vi "Speed Benchmark.vi"() -> ()   [LabVIEW 2015]
uses:
  <vilib>/Platform/TimedLoop/XDataNode/timing_clust.ctl
  <vilib>/Platform/TimedLoop/XDataNode/nitl_modes.ctl
  <vilib>/Platform/TimedLoop/XDataNode/wakeup.ctl
  <vilib>/rvi/Emulation/niFpgaSctlEmulationGetInTimedLoop.vi
  <vilib>/rvi/Emulation/niFpgaEmulationReportErrorSimple.vi
  <vilib>/rvi/Emulation/niFpgaGetClockAttributes.vi
  <vilib>/rvi/Emulation/niFpgaCriticalErrorInLSC.vi
  <vilib>/rvi/interface/RandomDataEmulation/niFpgaRandomDataHandleErrors.vi
  <vilib>/Platform/TimedLoop/XDataNode/XDataNode.xnode
  <vilib>/rvi/DataTransferAndStorage/Container/XNode/niFpgaContainer.xnode
  <vilib>/rvi/interface/RandomDataEmulation/nirviRandomDataFpgaReadWriteTemplate.vi
  <vilib>/Platform/TimedLoop/XDataNode/XDNodeRunTimeDep.lvlib
panel:
  out "Last index":i32
  out "First index":u32
  out "elements counter":u32
  out "TicksOut":u32
  in  "reset":bool
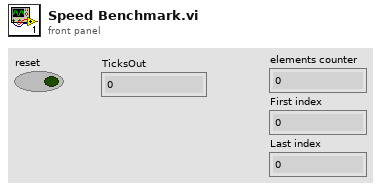
[diagram p1: front panel]
types:
  T1 = typedef "XDNodeRunTimeDep.lvlib/timing_clust.ctl" = cluster{"Expected End [f-1]":u64, "Actual End [f-1]":u64, "Finished Late? [f-1]":bool, "Expected End [i-1]":u64, "Actual End [i-1]":u64, "Finished Late? [i-1]":bool, "Expected Start [i]":u64, "Actual Start [i]":u64, "Expected Start [f]":u64, "Actual Start [f]":u64, "Source Name":string, "Structure Name":string, "Period":i64, "Deadline":i64, "Offset":i64, "Start":i64, "Priority":i32, "Timeout":i32, "Mode":T2, "Wakeup Reason":T3, "Error":errorcluster, "Source Type":string, "Secondary Source Type":string, "Global End Time":u64, "Global Start Time":u64, "Frame Duration":u64, "Iteration Duration":u64, "Assigned CPU":i32, "I/O Scan Engine Mode":u32}
  T2 = typedef "XDNodeRunTimeDep.lvlib/nitl_modes.ctl" = enum32{"No Change", "Process missed periods, maintain original phase", "Discard missed periods, maintain original phase", "Process missed periods, ignore original phase", "Discard missed periods, ignore original phase"}
  T3 = typedef "XDNodeRunTimeDep.lvlib/wakeup.ctl" = enum32{"Normal", "Aborted", "Asynchronous wakeup", "Timing source error", "Timed loop error", "Timeout"}
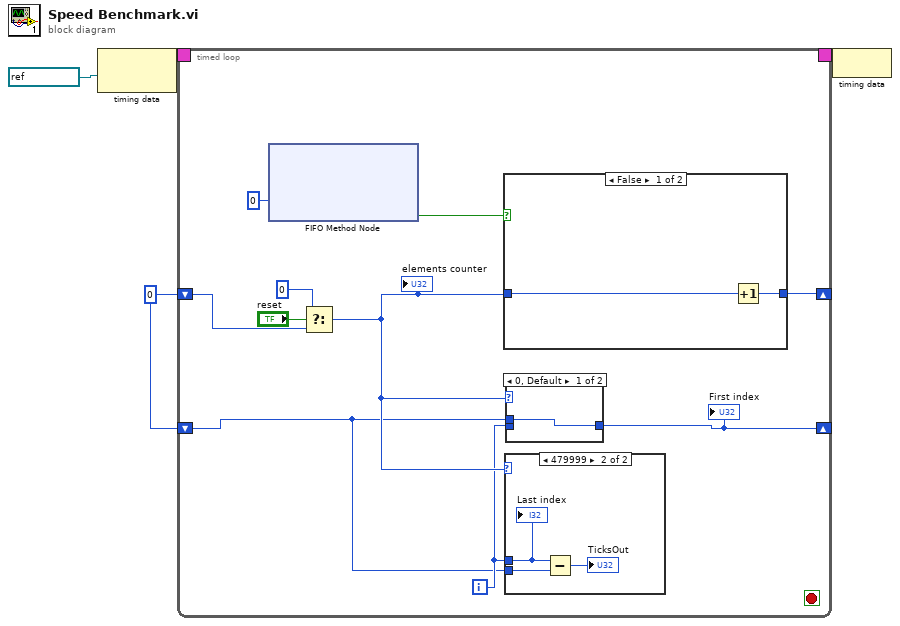
[diagram p0: block diagram]
diagram:
  w1 = u32 0
  n1 = node-c288(refnum<k21> "200MHz" ("Source Name")) -> (w4:T1)
  n2 = timed-loop {
    timing: w4 -> [_]
    timing-out: [_] -> w3
    shift-right: [w9] -> _
    shift-left: w1 -> [w11]
    shift-right: [w7] -> _
    shift-left: w1 -> [w5]
    i -> [w6]
    stop <- _ stop-if-true
    n3 = xnode ("FIFO Method Node")("Timeout"=0) -> ("Timed Out?"=w13:bool)  [unwired: 1 in, 2 out]
    n4 = Select(t=u32 0, s="reset", f=w11) -> (s? t:f=w8:u32)
    "elements counter" <- w8
    n5 = case shown="False" w13 {
      tunnel: w8 -> [w21 w22]
      tunnel: [w20 w22] -> w9
      frame False {
        n6 = Increment(x=w21) -> (x+1=w20:u32)
      }
      frame True {
      }
    }
    n7 = case shown="479999" w8 {
      tunnel: w6 -> [_ w17]
      tunnel: w5 -> [_ w16]
      frame 0, Default {
      }
      frame 479999 {
        n8 = Subtract(x=w17, y=w16) -> (x-y=→"TicksOut":u32)
        "Last index" <- w17
      }
    }
    n9 = case shown="0, Default" w8 {
      tunnel: w6 -> [_ w19]
      tunnel: [w18 w19] -> w7
      tunnel: w5 -> [w18 _]
      frame 0, Default {
      }
      frame 1 {
      }
    }
    "First index" <- w7
  }
  n10 = node-c288(w3) -> ()
